vi "PPMS.Status Ring to String.vi"(8 "error in (no error)":errorcluster, 9 "Field Status":T2 items=["MagnetUnknown"=0, "StablePersistent"=1, "WarmingSwitch"=2, "CoolingSwitch"=3, "StableDriven"=4, "Iterating"=5, "Charging"=6, "Discharging"=7, "CurrentError"=8, "MagnetFailure"=15], 10 "Temperature Status":T1 items=["TemperatureUnknown"=0, "Stable"=1, "Tracking"=2, "Near"=5, "Chasing"=6, "Filling"=7, "Standby"=10, "Disabled"=13, "ImpedanceNotFunction"=14, "TempFailure"=15], 11 "instrument.PPMS":refnum<class "instrument.PPMS.lvclass">) -> (0 "error out":errorcluster, 1 "Field Status String":string, 2 "Temperature Status String":string, 3 "instrument.PPMS out":refnum<class "instrument.PPMS.lvclass">)   [LabVIEW 2016, in "instrument.PPMS.lvclass"]
uses:
  instrument.PPMS.lvclass
  Typedefs/PPMS.Magnet Status--ring.ctl
  Typedefs/PPMS.Temperature Status--ring.ctl
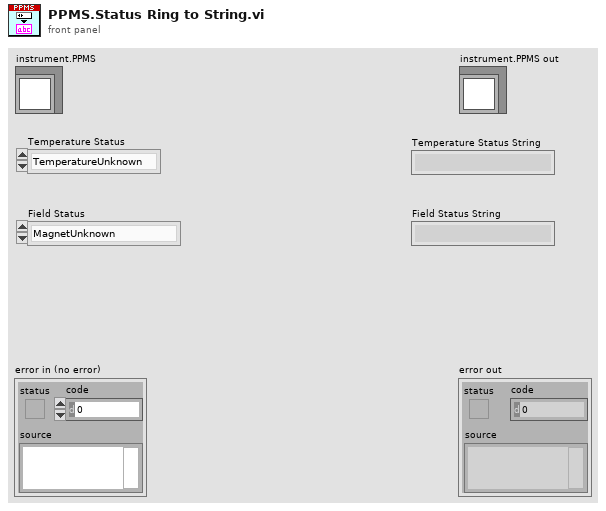
[diagram p1: front panel]
types:
  T1 = typedef "instrument.PPMS.lvclass/PPMS.Temperature Status--ring.ctl" = i32
  T2 = typedef "instrument.PPMS.lvclass/PPMS.Magnet Status--ring.ctl" = i32
  T3 = typedef "LVStringsAndValuesArrayTypeDef_I32.ctl" = cluster{"String":string, "Value":i32}[]
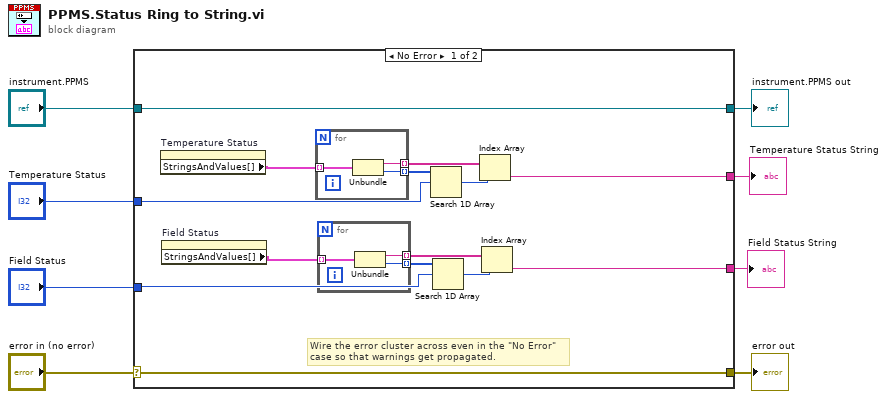
[diagram p0: block diagram]
diagram:
  n1 = case shown="No Error" "error in (no error)" {
    selector: "error in (no error)" -> [w21 w30]
    tunnel: [w21 w30] -> w7
    tunnel: [w22 w29] -> w5
    tunnel: "instrument.PPMS" -> [w22 w29]
    tunnel: "Temperature Status" -> [w19 _]
    tunnel: [w16 _] -> w4
    tunnel: "Field Status" -> [w12 _]
    tunnel: [w11 _] -> w3
    frame No Error {
      # "Wire the error cluster across even in the \"No Error\"\ncase so that warnings get propagated."
      n2 = property on="Temperature Status" class="Ring (strict)"() -> ("StringsAndValues[]"=w9:T3)  [unwired: 2 in, 2 out]
      n3 = property on="Field Status" class="Ring (strict)"() -> ("StringsAndValues[]"=w10:T3)  [unwired: 2 in, 2 out]
      n4 = for {
        tunnel: w9 -> [w28] mode=indexing
        tunnel: [w27] -> w20 mode=indexing
        tunnel: [w26] -> w17 mode=indexing
        n5 = Unbundle(w28) -> ("String"=w26:string, "Value"=w27:i32)
      }
      n6 = for {
        tunnel: w10 -> [w25] mode=indexing
        tunnel: [w24] -> w13 mode=indexing
        tunnel: [w23] -> w15 mode=indexing
        n7 = Unbundle(w25) -> ("String"=w23:string, "Value"=w24:i32)
      }
      n8 = Search 1D Array(1D array=w20, element=w19) -> (index of element=w18:i32)  [unwired: 1 in]
      n9 = Search 1D Array(1D array=w13, element=w12) -> (index of element=w14:i32)  [unwired: 1 in]
      n10 = Index Array(array=w17, index=w18) -> (element=w16:string)
      n11 = Index Array(array=w15, index=w14) -> (element=w11:string)
    }
    frame Error {
    }
  }
  "error out" <- w7
  "instrument.PPMS out" <- w5
  "Temperature Status String" <- w4
  "Field Status String" <- w3
